vi "up shift.vi"(11 "2048 2":dbl[][](array[numeric])) -> (3 "2048":dbl[][](array[numeric]))   [LabVIEW 2015]
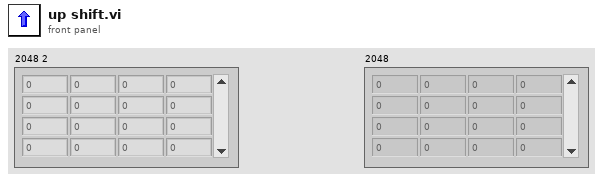
[diagram p1: front panel]
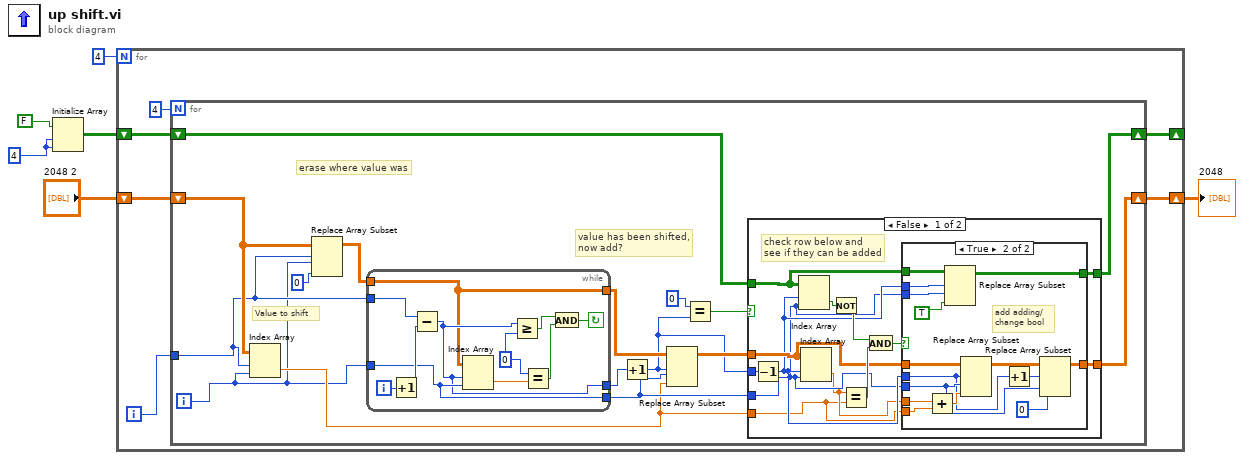
[diagram p0: block diagram]
diagram:
  w3 = 4
  n1 = Initialize Array(FALSE, w3, w3) -> (w1:bool[][])
  n2 = for {
    N: 4 -> [_]
    shift-right: [w8] -> _
    shift-left: w1 -> [w9]
    shift-right: [w7] -> w4
    shift-left: "2048 2" -> [w11]
    i -> [w10]
    n3 = for {
      N: 4 -> [_]
      tunnel: w10 -> [w14]
      shift-right: [w19] -> w8
      shift-left: w9 -> [w20]
      shift-right: [w18] -> w7
      shift-left: w11 -> [w16]
      i -> [w13]
      # "erase where value was"
      # "value has been shifted,\nnow add?"
      # "Value to shift"
      n4 = Index Array(array=w16, index (row)=w14, index (col)=w13) -> (element=w21:dbl)
      n5 = Replace Array Subset(array=w16, new element=0, index (row)=w14, index (col)=w13) -> (w17:dbl[][])
      n6 = while {
        tunnel: w14 -> [w71]
        tunnel: w13 -> [w63]
        tunnel: w17 -> [w61]
        tunnel: [w63] -> w24
        tunnel: [w62] -> w23
        tunnel: [w61] -> w28
        i -> [w70]
        stop <- w66 continue-if-true
        w65 = 0
        n7 = Increment(x=w70) -> (x+1=w67:i32)
        n8 = Subtract(x=w71, y=w67) -> (x-y=w62:i32)
        n9 = Index Array(array=w61, index (row)=w62, index (col)=w63) -> (element=w69:dbl)
        n10 = Greater Or Equal?(x=w62, y=w65) -> (x >= y?=w64:bool)
        n11 = Equal?(x=w65, y=w69) -> (x = y?=w68:bool)
        n12 = And(x=w64, y=w68) -> (x .and. y?=w66:bool)
      }
      n13 = Increment(x=w23) -> (x+1=w22:i32)
      n14 = Replace Array Subset(array=w28, new element=w21, index (row)=w22, index (col)=w24) -> (w25:dbl[][])
      n15 = Equal?(x=0, y=w22) -> (x = y?=w26:bool)
      n16 = case shown="False" w26 {
        tunnel: w25 -> [w35 w59]
        tunnel: w24 -> [w33 _]
        tunnel: w22 -> [w41 _]
        tunnel: w21 -> [w31 _]
        tunnel: w20 -> [w37 w60]
        tunnel: [w30 w60] -> w19
        tunnel: [w29 w59] -> w18
        frame False {
          # "check row below and \nsee if they can be added"
          n17 = Decrement(x=w41) -> (x-1=w34:i32)
          n18 = Index Array(array=w37, index (row)=w34, index (col)=w33) -> (element=w39:bool)
          n19 = Index Array(array=w35, index (row)=w34, index (col)=w33) -> (element=w32:dbl)
          n20 = Not(x=w39) -> (.not. x?=w38:bool)
          n21 = Equal?(x=w32, y=w31) -> (x = y?=w40:bool)
          n22 = And(x=w38, y=w40) -> (x .and. y?=w36:bool)
          n23 = case shown="True" w36 {
            tunnel: w37 -> [w43 w58]
            tunnel: w33 -> [_ w57]
            tunnel: w34 -> [_ w56]
            tunnel: w35 -> [w42 w54]
            tunnel: w34 -> [_ w45]
            tunnel: w33 -> [_ w46]
            tunnel: w32 -> [_ w52]
            tunnel: w31 -> [_ w51]
            tunnel: [w43 w50] -> w30
            tunnel: [w42 w48] -> w29
            frame False {
            }
            frame True {
              # "add adding/\nchange bool"
              n24 = Add(x=w52, y=w51) -> (x+y=w53:dbl)
              n25 = Replace Array Subset(array=w58, new element=TRUE, index (row)=w56, index (col)=w57) -> (w50:bool[][])
              n26 = Replace Array Subset(array=w54, new element=w53, index (row)=w45, index (col)=w46) -> (w49:dbl[][])
              n27 = Increment(x=w45) -> (x+1=w44:i32)
              n28 = Replace Array Subset(array=w49, new element=0, index (row)=w44, index (col)=w46) -> (w48:dbl[][])
            }
          }
        }
        frame True {
          # "if it is row 0 then,\n no adds to check"
        }
      }
    }
  }
  "2048" <- w4
